vi "setCurrentLimit.vi"(7 "chn":string, 8 "error in (no error)":errorcluster, 10 "currentLimit [A]":dbl, 11 "PsuNiPxi in":refnum<class "PsuNi.lvclass">) -> (0 "error out":errorcluster, 3 "PsuNiPxi out":refnum<class "PsuNi.lvclass">)   [LabVIEW 2023, in "PsuNi.lvclass"]
doc: "<b>Author:</b> Wolfgang\n<b>Description:</b> set output current limit of power supply by channel in A."
uses:
  PsuNi.lvclass
  PsuNi.lvclass/PsuNi.ctl
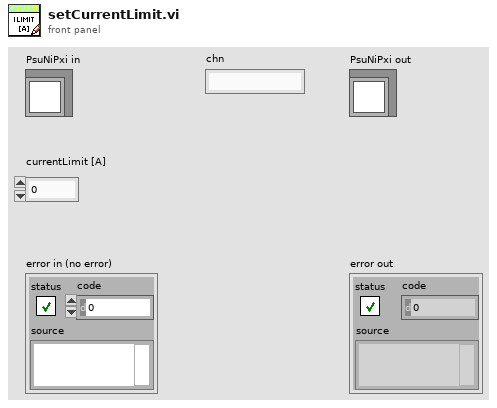
[diagram p1: front panel]
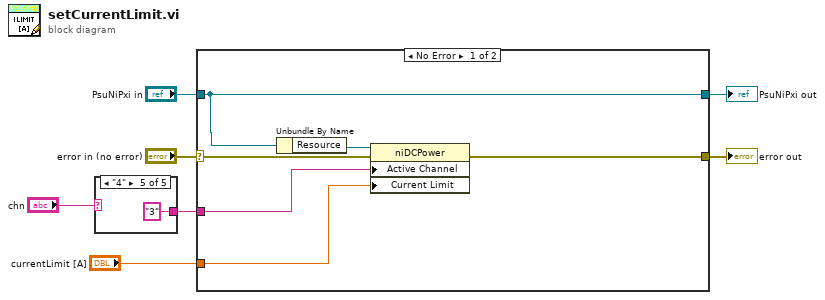
[diagram p0: block diagram]
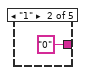
[diagram p3: hidden frame]
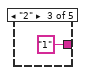
[diagram p4: hidden frame]
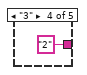
[diagram p5: hidden frame]
diagram:
  n1 = case shown="\"4\"" "chn" {
    selector: "chn" -> [w8 _ _ _ _]
    tunnel: [w8 "0" "1" "2" "3"] -> w1
    frame "False", Default {
    }
    frame "1" {
    }
    frame "2" {
    }
    frame "3" {
    }
    frame "4" {
    }
  }
  n2 = case shown="No Error" "error in (no error)" {
    selector: "error in (no error)" -> [w15 w19]
    tunnel: [w14 w19] -> w7
    tunnel: [w13 w20] -> w6
    tunnel: "PsuNiPxi in" -> [w13 w20]
    tunnel: w1 -> [w17 _]
    tunnel: "currentLimit [A]" -> [w16 _]
    frame No Error {
      n3 = Unbundle By Name(w13) -> ("Resource"=w18:refnum<k15>)
      n4 = property class="niDCPower"(reference=w18, error in=w15, "Active Channel"=w17, "Current Limit"=w16) -> (error out=w14:errorcluster)  [unwired: 1 out]
    }
    frame Error {
    }
  }
  "error out" <- w7
  "PsuNiPxi out" <- w6
